vi "Transcriptor LabVIEW to Python code Engine 3.vi"(7 "VI path":path, 8 "Error In":errorcluster, 10 "List Reentrant VIs":string[](array[string]), 11 "Diagram in":refnum<vi>) -> (0 "error out":errorcluster, 1 "output cluster":T1, 2 "transcripted code":string, 3 "Diagram out":refnum<vi>, 5 "VI ref.":refnum<vi>)   [LabVIEW 2014]
doc: "Transcript given Diagram or VI specified bz reference to Diagram or VI (one at time) to C++ code for Arduino platform. User must provide Diagram input or VI path input, transcripted code is available at output and also cluster with additional includes libraries string array and defines string array is available."
uses:
  types/LabVIEW Universal Transcriptor Cluster.ctl
  types/LabVIEW Universal Transcriptor C code Composer Input Cluster.ctl
  types/LabVIEW Universal Transcriptor Structure Definitions.ctl
panel:
  out "FiringOrder":string[](array[string])
  # "0. create definitions (ClusterConstant)\n1. get all wires and create their declarations\n2. if wires are connected to control or constant assign value to them\n3. translate elements of diagram by firing order\n4. assign values to outputs"
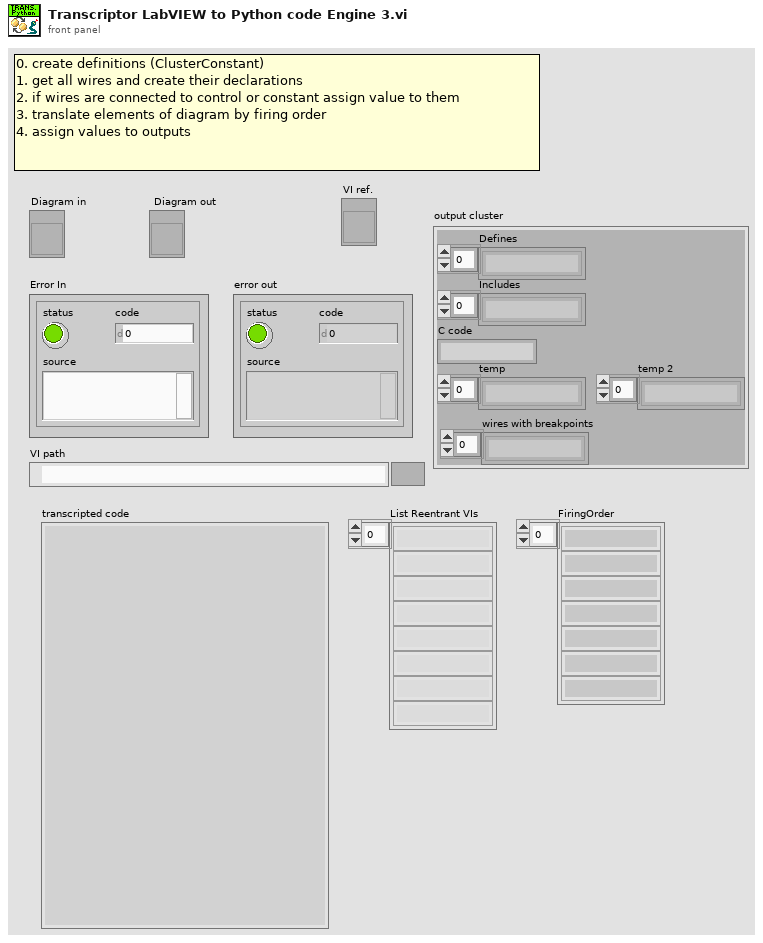
[diagram p1: front panel]
types:
  T1 = typedef "LabVIEW Universal Transcriptor Cluster.ctl" = cluster{"Defines":string[], "Includes":string[], "C code":string, "temp":string[], "temp 2":string[], "wires with breakpoints":string[]}
  T2 = typedef "LabVIEW Universal Transcriptor C code Composer Input Cluster.ctl" = cluster{"structure definitions cluster":T3, "end loop refs.":string[], "wires declarations":string[], "diagram ref.":refnum<vi>, "transcriptor cluster":T1[], "transcripted C code":string[], "output value assignement":string, "feedbackNodes assignements":string[], "wires with breakpoints":string[]}
  T3 = typedef "LabVIEW Universal Transcriptor Structure Definitions.ctl" = cluster{"Cluster def.":string[], "FeedbacNode def.":string[], "ShiftReg def.":string[]}
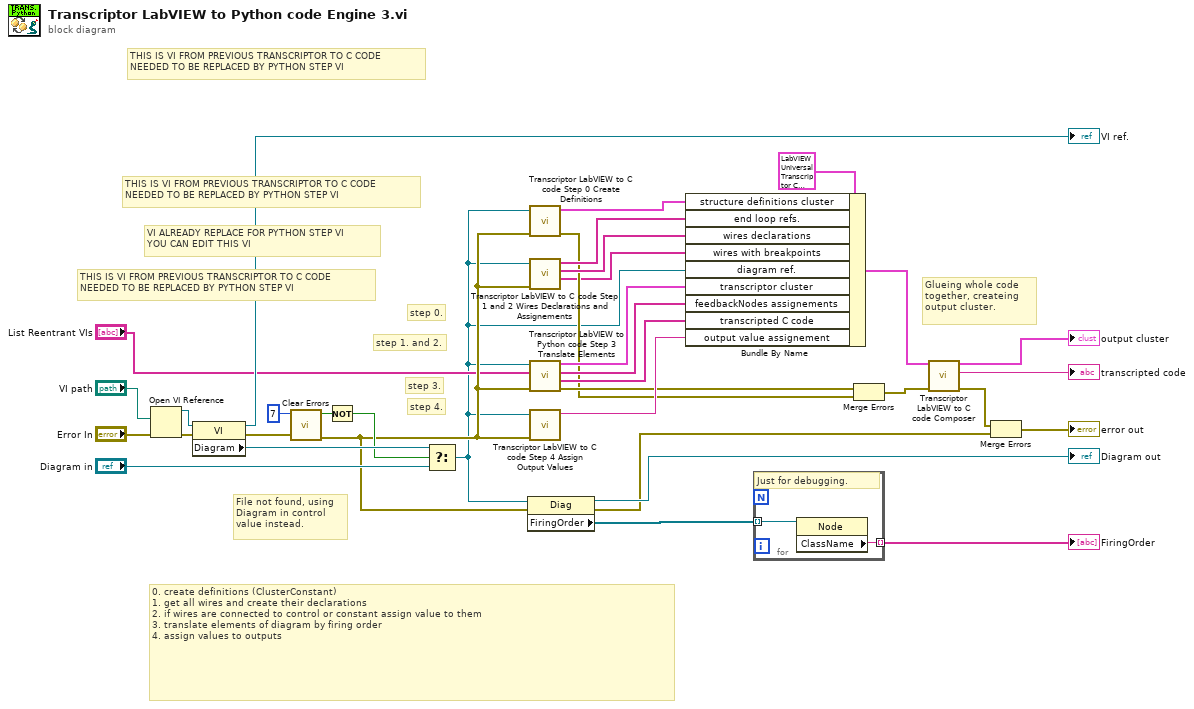
[diagram p0: block diagram]
diagram:
  # "VI ALREADY REPLACE FOR PYTHON STEP VI\nYOU CAN EDIT THIS VI"
  # "THIS IS VI FROM PREVIOUS TRANSCRIPTOR TO C CODE\nNEEDED TO BE REPLACED BY PYTHON STEP VI"
  # "THIS IS VI FROM PREVIOUS TRANSCRIPTOR TO C CODE\nNEEDED TO BE REPLACED BY PYTHON STEP VI"
  # "THIS IS VI FROM PREVIOUS TRANSCRIPTOR TO C CODE\nNEEDED TO BE REPLACED BY PYTHON STEP VI"
  # "Glueing whole code together, createing output cluster."
  # "step 4."
  # "step 3."
  # "step 1. and 2."
  # "step 0."
  # "0. create definitions (ClusterConstant)\n1. get all wires and create their declarations\n2. if wires are connected to control or constant assign value to them\n3. translate elements of diagram by firing order\n4. assign values to outputs"
  # "File not found, using Diagram in control value instead."
  n1 = Open VI Reference(vi path="VI path", error in (no error)="Error In") -> (vi reference=w27:refnum<vi>, error out=w34:errorcluster)  [unwired: 4 in]
  n2 = property on="Property Node" class="VI"(reference=w27, error in=w34) -> (reference out=→"VI ref.":refnum<vi>, error out=w6:errorcluster, "Diagram"=w33:refnum<vi>)
  n3 = call <vilib>:"Clear Errors.vi"("error in (no error)"=w6, "specific error code to clear (0: all)"=7) -> ("error out"=w7:errorcluster, "specific error cleared?"=w30:bool)  [unwired: 4 in]
  n4 = Not(x=w30) -> (.not. x?=w29:bool)
  n5 = Select(t=w33, s=w29, f="Diagram in") -> (s? t:f=w2:refnum<vi>)
  n6 = property on="Property Node" class="Diag"(reference=w2, error in=w7) -> (reference out=→"Diagram out":refnum<vi>, error out=w11:errorcluster, "FiringOrder"=w25:refnum<vi>[])
  n7 = call "Transcriptor LabVIEW to C code Step 0 Create Definitions.vi"("error in"=w7, "Diagram in"=w2) -> ("error out"=w8:errorcluster, "structure definition cluster"=w3:T3)  [unwired: 8 in]
  n8 = call "Transcriptor LabVIEW to C code Step 1 and 2 Wires Declarations and Assignements.vi"("error in"=w7, "Diagram in"=w2) -> ("wires with enabled breakpoints"=w1:string[], "wires declarations"=w19:string[], "end loop refs."=w20:string[])  [unwired: 7 in]
  n9 = call "Transcriptor LabVIEW to Python code Step 3 Translate Elements.vi"("error in (no error)"=w7, "reentrant VIs"="List Reentrant VIs", "Diagram in"=w2) -> ("error out"=w9:errorcluster, "transcripted C code"=w16:string[], "feedback assignments"=w17:string[], "transcriptor cluster"=w18:T1[])  [unwired: 5 in]
  n10 = call "Transcriptor LabVIEW to C code Step 4 Assign Output Values.vi"("error in (no error)"=w7, "Diagram in"=w2) -> ("output value assignement"=w15:string)  [unwired: 9 in]
  n11 = Bundle By Name(cluster=T2 {"structure definitions cluster"={"Cluster def."=[], "FeedbacNode def."=[], "ShiftReg def."=[]}, "end loop refs."=[], "wires declarations"=[], "diagram ref."=refnum, "transcriptor cluster"=[], "transcripted C code"=[], "output value assignement"="", "feedbackNodes assignements"=[], "wires with breakpoints"=[]} ("Cluster"), "structure definitions cluster"=w3, "end loop refs."=w20, "wires declarations"=w19, "wires with breakpoints"=w1, "diagram ref."=w2, "transcriptor cluster"=w18, "feedbackNodes assignements"=w17, "transcripted C code"=w16, "output value assignement"=w15) -> (w22:T2)
  n12 = for {
    tunnel: w25 -> [w37] mode=indexing
    tunnel: [w36] -> w32 mode=indexing
    # "Just for debugging."
    n13 = property class="Node"(reference=w37) -> ("ClassName"=w36:string)  [unwired: 1 in, 2 out]
  }
  "FiringOrder" <- w32
  n14 = Merge Errors(w9, w8) -> (w10:errorcluster)
  n15 = call "Transcriptor LabVIEW to C code Composer.vi"("error in (no error)"=w10, "C code Composer Cluster in"=w22) -> ("error out"=w13:errorcluster, "transcripted code"=→"transcripted code":string, "output cluster"=→"output cluster":T1)  [unwired: 7 in]
  n16 = Merge Errors(w13, w11) -> (→"error out":errorcluster)
